vi "set_calibration.vi"(5 "y unit":T1, 7 "x unit":T1, 8 "error in (no error)":errorcluster, 9 "y":dbl, 10 "x":dbl, 11 "DL090211ImageAssemblerScaffold in":refnum<class "ImageAssemblerDL090211Scaffold.lvclass">) -> (0 "error out":errorcluster, 3 "DL090211ImageAssemblerScaffold out":refnum<class "ImageAssemblerDL090211Scaffold.lvclass">)   [LabVIEW 2010, in "ImageAssemblerDL090211Scaffold.lvclass"]
uses:
  ImageAssemblerDL090211Scaffold.lvclass
  common/enumerations/unit.ctl
  ImageAssemblerDL090211Scaffold.lvclass/ImageAssemblerDL090211Scaffold.ctl
  common/classes/Image/Image/Image.lvclass
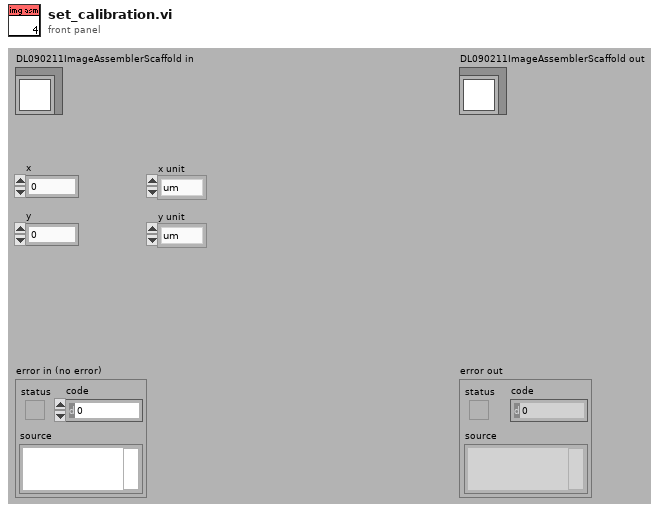
[diagram p1: front panel]
types:
  T1 = typedef "Image.lvclass/unit.ctl" = enum16{"um", "s"}
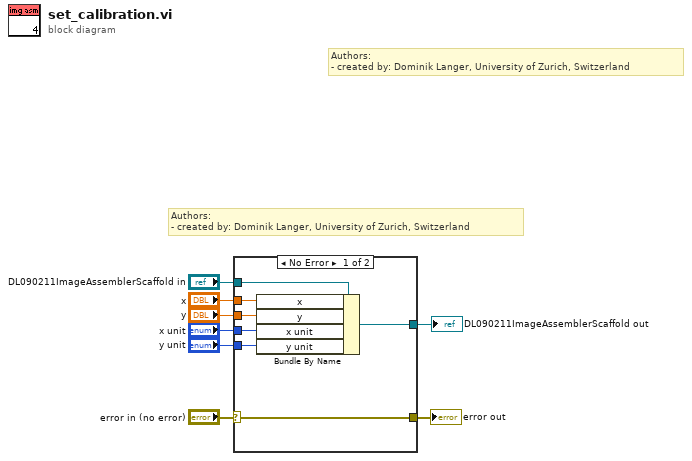
[diagram p0: block diagram]
diagram:
  # "Authors: \n- created by: Dominik Langer, University of Zurich, Switzerland"
  # "Authors: \n- created by: Dominik Langer, University of Zurich, Switzerland"
  n1 = case shown="No Error" "error in (no error)" {
    selector: "error in (no error)" -> [w13 w17]
    tunnel: [w13 w17] -> w7
    tunnel: [w15 w16] -> w5
    tunnel: "DL090211ImageAssemblerScaffold in" -> [w14 w16]
    tunnel: "x" -> [w10 _]
    tunnel: "y" -> [w9 _]
    tunnel: "x unit" -> [w11 _]
    tunnel: "y unit" -> [w12 _]
    frame No Error {
      n2 = Bundle By Name(cluster=w14, "x"=w10, "y"=w9, "x unit"=w11, "y unit"=w12) -> (w15:refnum<class "ImageAssemblerDL090211Scaffold.lvclass">)
    }
    frame Error {
    }
  }
  "error out" <- w7
  "DL090211ImageAssemblerScaffold out" <- w5
